vi "getunionRect.vi"(8 "error in (no error)":errorcluster, 11 "GObjects":refnum<class "GObject.lvclass">[](array[class])) -> (0 "error out":errorcluster, 2 "unionRect":T1, 3 "GObjects(dup)":refnum<class "GObject.lvclass">[](array[class]))   [LabVIEW 2023, in "TLC_Scripto.lvlib"]
uses:
  GObject/GObject.lvclass
  Ctrls/rectangle.ctl
  TLC_Scripto.lvlib
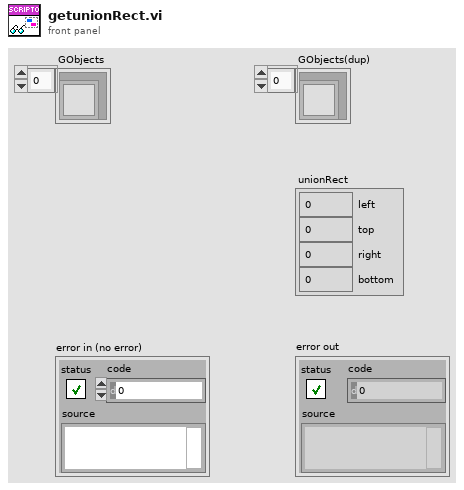
[diagram p1: front panel]
types:
  T1 = typedef "TLC_Scripto.lvlib/rectangle.ctl" = cluster{"left":i32, "top":i32, "right":i32, "bottom":i32}
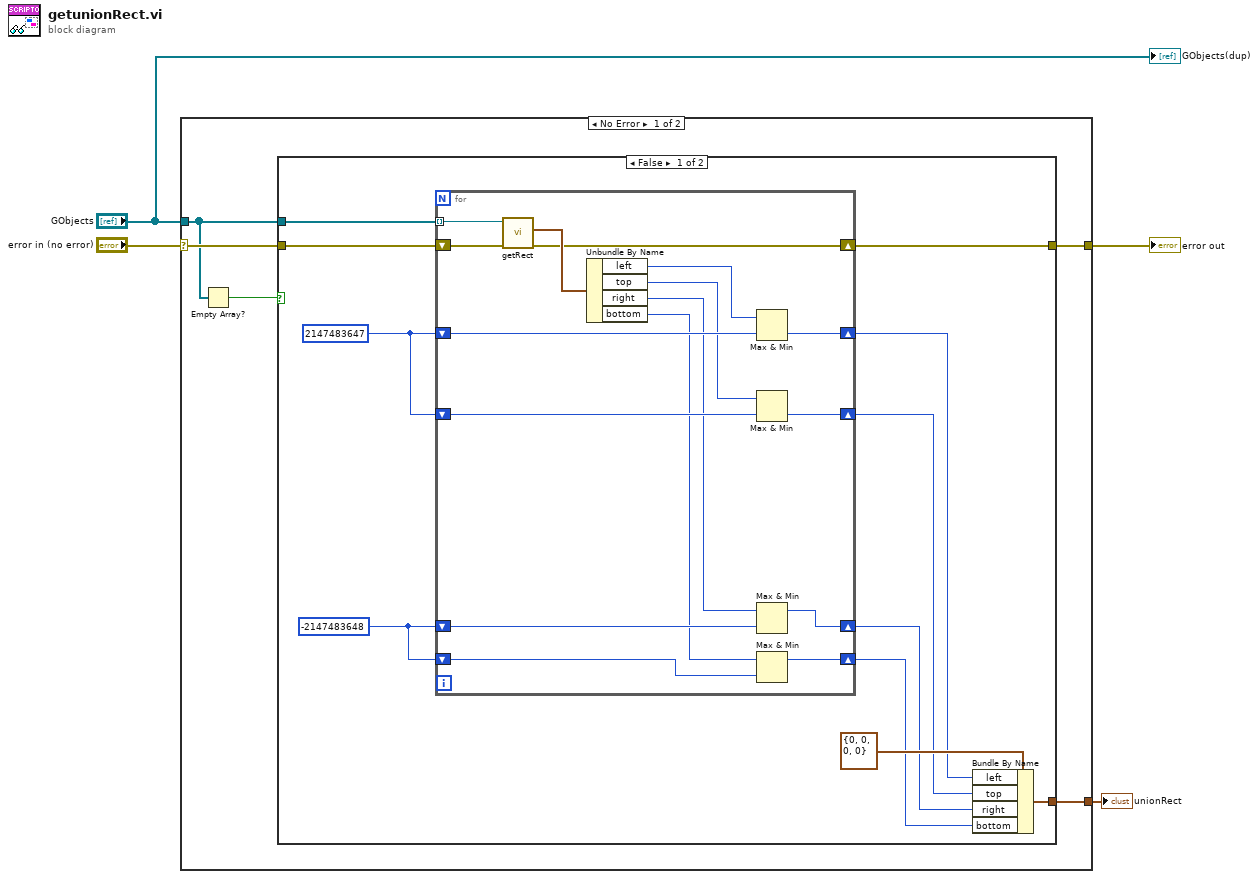
[diagram p0: block diagram]
diagram:
  n1 = case shown="No Error" "error in (no error)" {
    selector: "error in (no error)" -> [w8 w38]
    tunnel: "GObjects" -> [w6 _]
    tunnel: [w7 w38] -> w3
    tunnel: [w9 _] -> w1
    frame No Error {
      n2 = Empty Array?(array=w6) -> (empty?=w5:bool)
      n3 = case shown="False" w5 {
        tunnel: [w14 _] -> w9
        tunnel: w8 -> [w13 w37]
        tunnel: [w12 w37] -> w7
        tunnel: w6 -> [w11 _]
        frame False {
          w10 = -2147483648
          w20 = 2147483647
          n4 = for {
            tunnel: w11 -> [w36] mode=indexing
            shift-right: [w33] -> w18
            shift-left: w20 -> [w32]
            shift-right: [w29] -> w17
            shift-left: w20 -> [w30]
            shift-right: [w25] -> w16
            shift-left: w10 -> [w27]
            shift-right: [w24] -> w15
            shift-left: w10 -> [w23]
            shift-right: [w21] -> w12
            shift-left: w13 -> [w22]
            n5 = call-dynamic "getRect.vi"("error in (no error)"=w22, "GObject in"=w36) -> ("error out"=w21:errorcluster, "rectangle"=w35:T1)  [unwired: 7 in, 1 out]
            n6 = Unbundle By Name(w35) -> ("left"=w34:i32, "top"=w31:i32, "right"=w28:i32, "bottom"=w26:i32)
            n7 = Max & Min(x=w34, y=w32) -> (min(x,y)=w33:i32)  [unwired: 1 out]
            n8 = Max & Min(x=w31, y=w30) -> (min(x,y)=w29:i32)  [unwired: 1 out]
            n9 = Max & Min(x=w28, y=w27) -> (max(x,y)=w25:i32)  [unwired: 1 out]
            n10 = Max & Min(x=w26, y=w23) -> (max(x,y)=w24:i32)  [unwired: 1 out]
          }
          n11 = Bundle By Name(cluster=T1 {"left"=0, "top"=0, "right"=0, "bottom"=0} ("rectangle"), "left"=w18, "top"=w17, "right"=w16, "bottom"=w15) -> (w14:T1)
        }
        frame True {
        }
      }
    }
    frame Error {
    }
  }
  "error out" <- w3
  "unionRect" <- w1
  "GObjects(dup)" <- "GObjects"
